vi "DriveModuleNetwork.vi"(8 "error in (no error)":errorcluster, 11 "Module":i32) -> (0 "error out":errorcluster)   [LabVIEW 2023]
doc: "Network for Drive\n\nInputs:\n -- Error in -- Error cluster -- propagated error input\n\nOutputs:\n -- Error out -- Error cluster -- progated error output"
uses:
  DriveGlobal.vi
  <vilib>/Rock Robotics/Network Tables/NT Write Number.vi
  <vilib>/Rock Robotics/WPI/ThirdParty/JAS_Junk/TrajLib/Trajectory_Library.lvlib
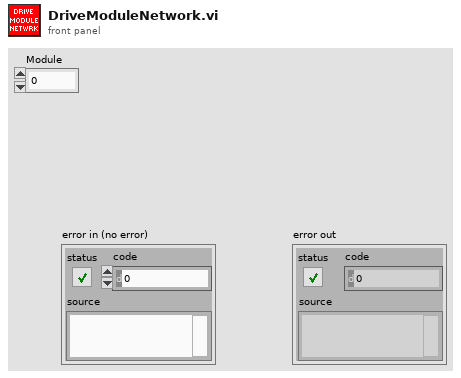
[diagram p1: front panel]
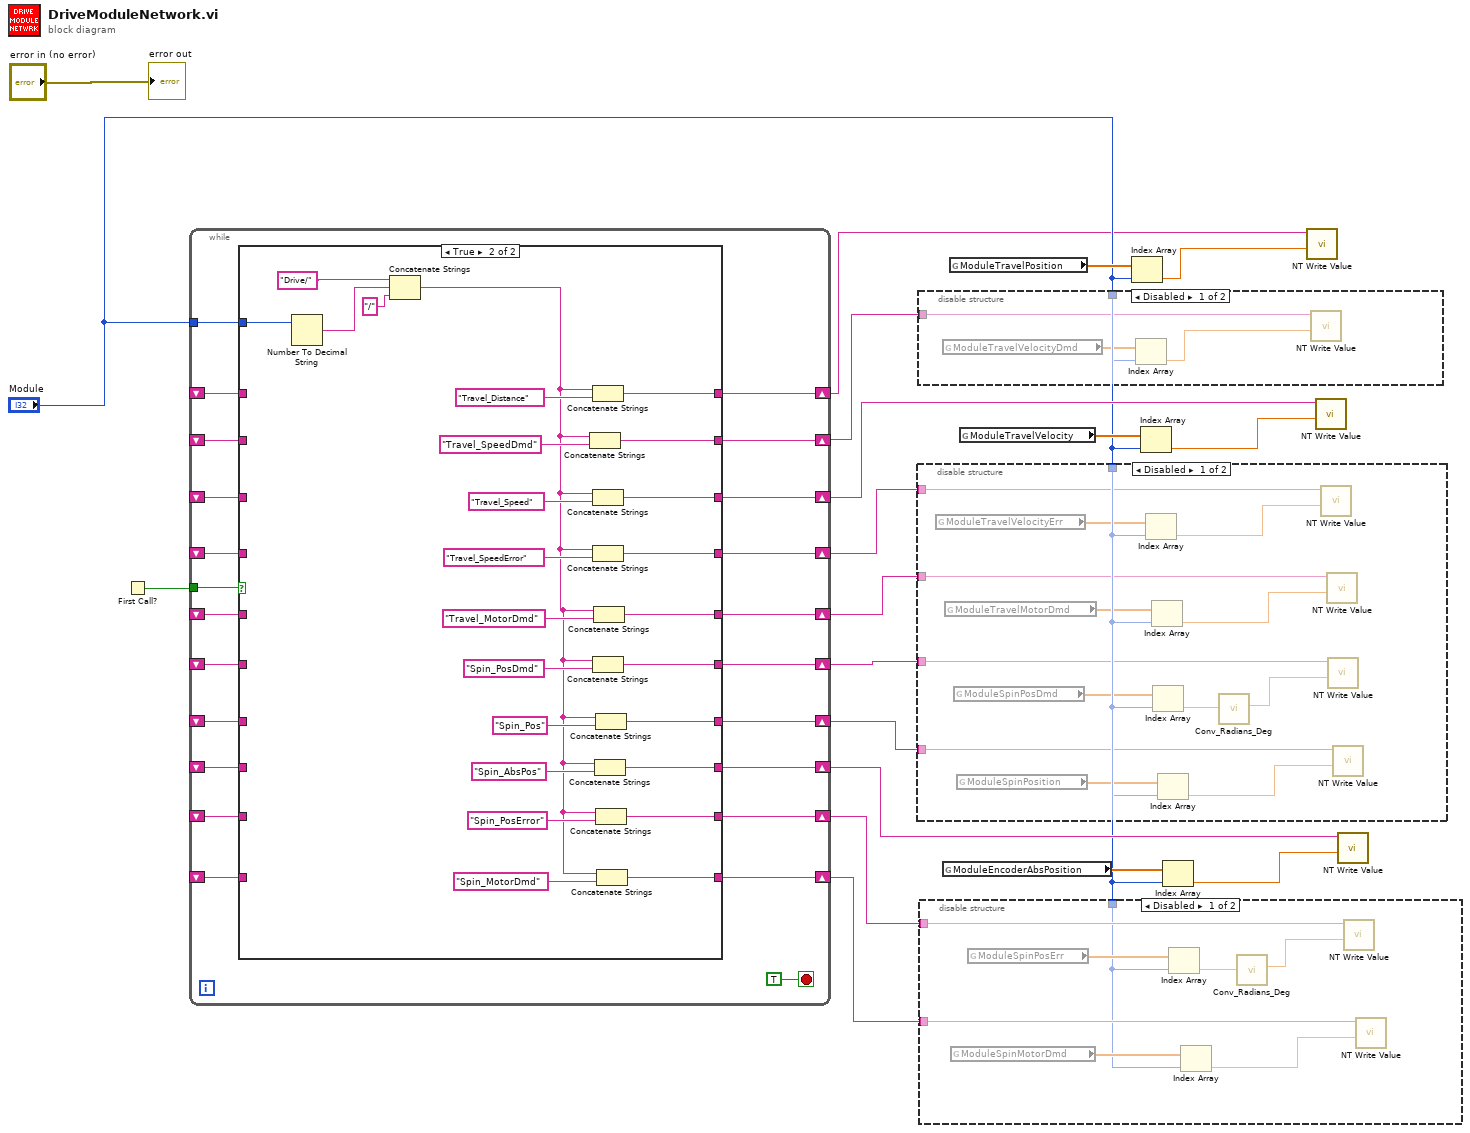
[diagram p0: block diagram]
diagram:
  n1 = First Call?() -> (First Call?: T/F=w18:bool)
  n2 = while {
    tunnel: w18 -> [w41]
    tunnel: "Module" -> [w40]
    shift-right: [w39] -> w17
    shift-left: _ -> [w30]
    shift-right: [w38] -> w12
    shift-left: _ -> [w29]
    shift-right: [w37] -> w11
    shift-left: _ -> [w27]
    shift-right: [w36] -> w10
    shift-left: _ -> [w28]
    shift-right: [w35] -> w9
    shift-left: _ -> [w26]
    shift-right: [w34] -> w8
    shift-left: _ -> [w25]
    shift-right: [w33] -> w7
    shift-left: _ -> [w24]
    shift-right: [w32] -> w6
    shift-left: _ -> [w23]
    shift-right: [w31] -> w5
    shift-left: _ -> [w22]
    shift-right: [w21] -> w1
    shift-left: _ -> [w20]
    stop <- TRUE stop-if-true
    n3 = case shown="True" w41 {
      tunnel: w40 -> [_ w76]
      tunnel: [w52 w64] -> w39
      tunnel: [w51 w63] -> w38
      tunnel: [w49 w62] -> w37
      tunnel: [w50 w61] -> w36
      tunnel: [w48 w60] -> w35
      tunnel: [w47 w59] -> w34
      tunnel: [w46 w58] -> w33
      tunnel: [w45 w57] -> w32
      tunnel: [w44 w56] -> w31
      tunnel: w30 -> [w52 _]
      tunnel: w29 -> [w51 _]
      tunnel: w28 -> [w50 _]
      tunnel: w27 -> [w49 _]
      tunnel: w26 -> [w48 _]
      tunnel: w25 -> [w47 _]
      tunnel: w24 -> [w46 _]
      tunnel: w23 -> [w45 _]
      tunnel: w22 -> [w44 _]
      tunnel: [w43 w53] -> w21
      tunnel: w20 -> [w43 _]
      frame False {
      }
      frame True {
        n4 = Number To Decimal String(number=w76) -> (decimal integer string=w75:string)  [unwired: 1 in]
        n5 = Concatenate Strings("Drive/", w75, "/" ("string")) -> (w54:string)
        n6 = Concatenate Strings(w54, "Travel_SpeedDmd" ("string")) -> (w64:string)
        n7 = Concatenate Strings(w54, "Travel_Distance" ("string")) -> (w53:string)
        n8 = Concatenate Strings(w54, "Travel_Speed" ("string")) -> (w63:string)
        n9 = Concatenate Strings(w54, "Travel_SpeedError" ("string")) -> (w62:string)
        n10 = Concatenate Strings(w54, "Spin_PosDmd" ("string")) -> (w60:string)
        n11 = Concatenate Strings(w54, "Travel_MotorDmd" ("string")) -> (w61:string)
        n12 = Concatenate Strings(w54, "Spin_AbsPos" ("string")) -> (w58:string)
        n13 = Concatenate Strings(w54, "Spin_Pos" ("string")) -> (w59:string)
        n14 = Concatenate Strings(w54, "Spin_PosError" ("string")) -> (w57:string)
        n15 = Concatenate Strings(w54, "Spin_MotorDmd" ("string")) -> (w56:string)
      }
    }
  }
  n16 = disable-structure shown="Disabled" {
    disable-tunnel: w11 -> [w84 _]
    disable-tunnel: w10 -> [w83 _]
    disable-tunnel: w9 -> [w82 _]
    disable-tunnel: w8 -> [w81 _]
    disable-tunnel: "Module" -> [w80 _]
    frame Disabled {
      n17 = global read "DriveGlobal.vi" "ModuleTravelVelocityErr"() -> (w91:dbl[])
      n18 = global read "DriveGlobal.vi" "ModuleTravelMotorDmd"() -> (w89:dbl[])
      n19 = global read "DriveGlobal.vi" "ModuleSpinPosDmd"() -> (w87:dbl[])
      n20 = global read "DriveGlobal.vi" "ModuleSpinPosition"() -> (w86:dbl[])
      n21 = Index Array(array=w91, index=w80) -> (element=w90:dbl)
      n22 = Index Array(array=w89, index=w80) -> (element=w88:dbl)
      n23 = Index Array(array=w87, index=w80) -> (element=w79:dbl)
      n24 = Index Array(array=w86, index=w80) -> (element=w85:dbl)
      n25 = call <vilib>:"Conv_Radians_Deg.vi"("Radians"=w79) -> ("Degrees"=w78:dbl)  [unwired: 10 in]
      n26 = call-poly <vilib>:"NT Write Value.vi"("value"=w90, "name"=w84) -> ()  [unwired: 9 in, 1 out]
      n27 = call-poly <vilib>:"NT Write Value.vi"("value"=w88, "name"=w83) -> ()  [unwired: 9 in, 1 out]
      n28 = call-poly <vilib>:"NT Write Value.vi"("value"=w78, "name"=w82) -> ()  [unwired: 9 in, 1 out]
      n29 = call-poly <vilib>:"NT Write Value.vi"("value"=w85, "name"=w81) -> ()  [unwired: 9 in, 1 out]
    }
    frame Enabled {
    }
  }
  n30 = disable-structure shown="Disabled" {
    disable-tunnel: w17 -> [w95 _]
    disable-tunnel: "Module" -> [w92 _]
    frame Disabled {
      n31 = global read "DriveGlobal.vi" "ModuleTravelVelocityDmd"() -> (w94:dbl[])
      n32 = Index Array(array=w94, index=w92) -> (element=w93:dbl)
      n33 = call-poly <vilib>:"NT Write Value.vi"("value"=w93, "name"=w95) -> ()  [unwired: 9 in, 1 out]
    }
    frame Enabled {
    }
  }
  n34 = disable-structure shown="Disabled" {
    disable-tunnel: w6 -> [w100 _]
    disable-tunnel: w5 -> [w99 _]
    disable-tunnel: "Module" -> [w98 _]
    frame Disabled {
      n35 = global read "DriveGlobal.vi" "ModuleSpinMotorDmd"() -> (w102:dbl[])
      n36 = global read "DriveGlobal.vi" "ModuleSpinPosErr"() -> (w103:dbl[])
      n37 = Index Array(array=w103, index=w98) -> (element=w97:dbl)
      n38 = Index Array(array=w102, index=w98) -> (element=w101:dbl)
      n39 = call <vilib>:"Conv_Radians_Deg.vi"("Radians"=w97) -> ("Degrees"=w96:dbl)  [unwired: 10 in]
      n40 = call-poly <vilib>:"NT Write Value.vi"("value"=w96, "name"=w100) -> ()  [unwired: 9 in, 1 out]
      n41 = call-poly <vilib>:"NT Write Value.vi"("value"=w101, "name"=w99) -> ()  [unwired: 9 in, 1 out]
    }
    frame Enabled {
    }
  }
  n42 = global read "DriveGlobal.vi" "ModuleEncoderAbsPosition"() -> (w14:dbl[])
  n43 = global read "DriveGlobal.vi" "ModuleTravelPosition"() -> (w4:dbl[])
  n44 = global read "DriveGlobal.vi" "ModuleTravelVelocity"() -> (w16:dbl[])
  n45 = Index Array(array=w4, index="Module") -> (element=w3:dbl)
  n46 = Index Array(array=w16, index="Module") -> (element=w15:dbl)
  n47 = Index Array(array=w14, index="Module") -> (element=w13:dbl)
  n48 = call-poly <vilib>:"NT Write Value.vi"("value"=w3, "name"=w1) -> ()  [unwired: 9 in, 1 out]
  n49 = call-poly <vilib>:"NT Write Value.vi"("value"=w15, "name"=w12) -> ()  [unwired: 9 in, 1 out]
  n50 = call-poly <vilib>:"NT Write Value.vi"("value"=w13, "name"=w7) -> ()  [unwired: 9 in, 1 out]
  "error out" <- "error in (no error)"
